vi "Example7.vi"() -> ()   [LabVIEW 2019]
panel:
  out "I":dbl
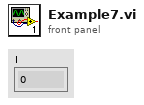
[diagram p1: front panel]
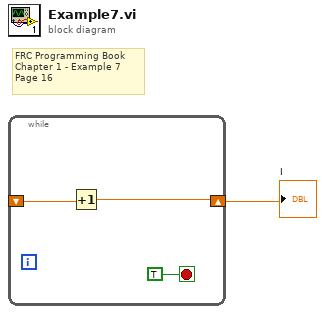
[diagram p0: block diagram]
diagram:
  # "FRC Programming Book\nChapter 1 - Example 7\nPage 16"
  n1 = while {
    shift-right: [w2] -> w1
    shift-left: _ -> [w3]
    stop <- TRUE stop-if-true
    n2 = Increment(x=w3) -> (x+1=w2:dbl)
  }
  "I" <- w1
